vi "Test_Plot_Name.vi"() -> ()   [LabVIEW 2013]
panel:
  in  "Nom des traces":string[](array[string])
  out "Graphe déroulant":dbl(graph)
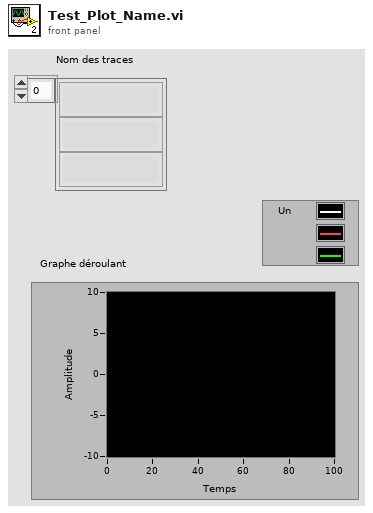
[diagram p1: front panel]
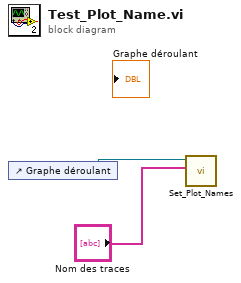
[diagram p0: block diagram]
diagram:
  n1 = control-ref of="Graphe déroulant"() -> (w2:refnum<vi>)
  n2 = call "Set_Plot_Names.vi"("Nom des traces"="Nom des traces", "Ref au graphe"=w2) -> ()  [unwired: 8 in, 1 out]
